vi "UIRef.vi"(8 "error in":errorcluster, 11 "Polynomial Scale editor node in":refnum<class "Polynomial Scale editor node.lvclass">) -> (0 "error out":errorcluster, 2 "VI refnum":refnum<vi>, 3 "Polynomial Scale editor node out":refnum<class "Polynomial Scale editor node.lvclass">)   [LabVIEW 2013]
uses:
  Polynomial Scale editor node.lvclass
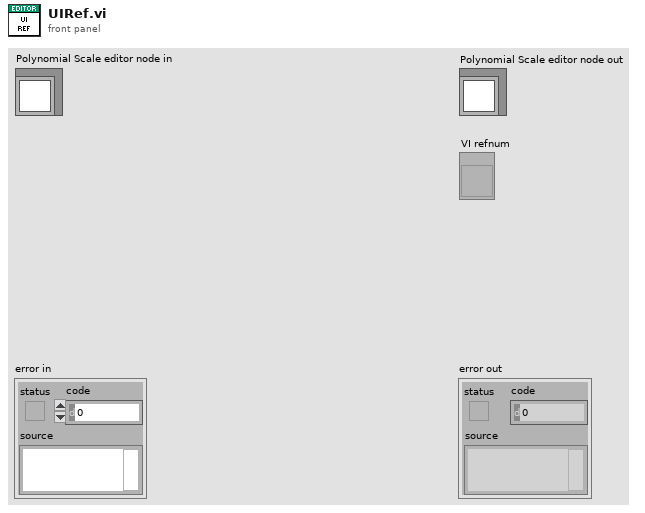
[diagram p1: front panel]
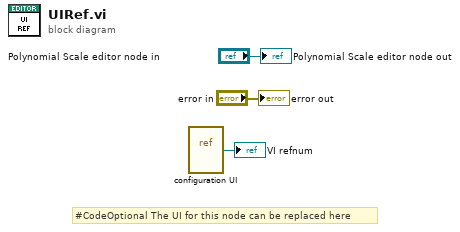
[diagram p0: block diagram]
diagram:
  # "#CodeOptional The UI for this node can be replaced here"
  n1 = vi-ref "configuration UI.vi"() -> (→"VI refnum":refnum<vi>)
  "error out" <- "error in"
  "Polynomial Scale editor node out" <- "Polynomial Scale editor node in"
